vi "Call Async Do.vi"(10 "Async Methods Actor in":refnum<class "Async Methods Actor.lvclass">, 11 "Message in":refnum<class "Message.lvclass">) -> (0 "error out":errorcluster, 2 "Async Methods Actor out":refnum<class "Async Methods Actor.lvclass">)   [LabVIEW 2021, in "Async Methods Actor.lvlib" / "Async Methods Actor.lvclass"]
uses:
  Async Methods Actor.lvclass
  <vilib>/ActorFramework/Message/Message.lvclass
  C:/Program Files/National Instruments/LabVIEW 2021/vi.lib/ActorFramework/Actor/Actor.lvclass
  Async Methods Actor.lvclass/Async Methods Actor.ctl
  VI Refnums Map Value.ctl
  Async Call Method.ctl
  VI Refnum Lifetime.ctl
  Async Methods Actor Messages/Async Message/Async Message.lvclass
  Async Methods Actor Messages/Async Message/Async Message.lvclass/Async Message.ctl
  Async Methods Actor Messages/Async Message/Read Async Call Method.vi
  Async Methods Actor Messages/Async Message/Read VI Refnum Lifetime.vi
  Write Async Message Execution Status Map.vi
  Async Methods Actor Messages/Async Message/Read FQN.vi
  Write Async Message Execution Status Map.vi/3adbf29e-89d7-4ecb-a2bd-8a8b89d527f8.vi
  Get VI FQN.vi
  <vilib>/ActorFramework/Actor/Actor.lvclass
  C:/Projects/Async Methods Actor/Async Methods Actor/Async Methods Actor/Async Methods Actor.lvclass
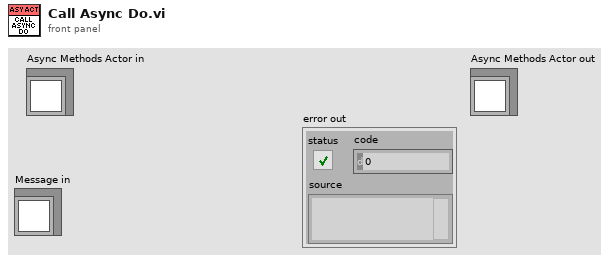
[diagram p1: front panel]
types:
  T1 = typedef "Async Methods Actor.lvlib/Async Methods Actor.lvclass/VI Refnums Map Value.ctl" = cluster{"Async Call Method":T2, "VI Refnum Lifecycle":T3, "Message Path":path}
  T2 = typedef "Async Methods Actor.lvlib/Async Methods Actor.lvclass/Async Call Method.ctl" = enum16{"Call and Collect", "Call and Forget"}
  T3 = typedef "Async Methods Actor.lvlib/Async Methods Actor.lvclass/VI Refnum Lifetime.ctl" = enum16{"Destroy on Exit", "Destroy on Actor Exit", "Leak"}
  T4 = typedef "Async Methods Actor.lvlib/Async Methods Actor.lvclass/VI Refnums Map.ctl" = map{refnum<vi>, T1}
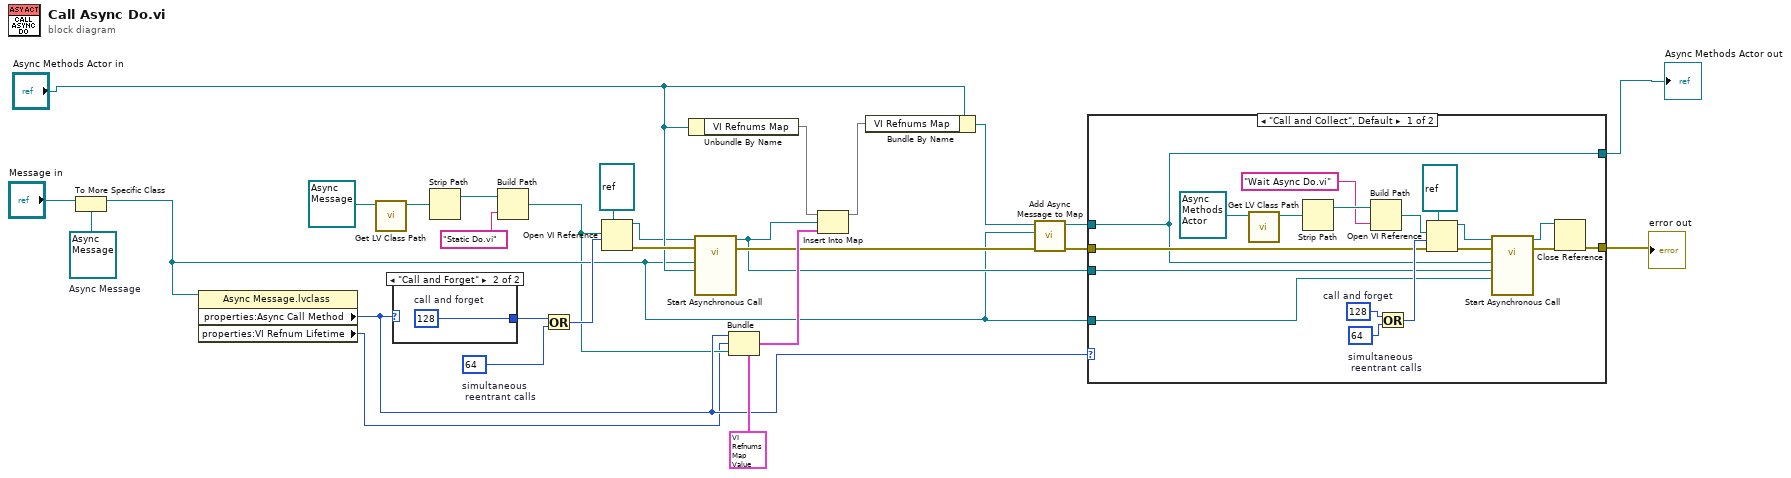
[diagram p0: block diagram]
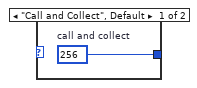
[diagram p3: hidden frame]
diagram:
  w25 = refnum<class "Async Message.lvclass"> refnum  # Async Message
  w23 = 64  # simultaneous  reentrant calls
  n1 = To More Specific Class(target class=w25, reference="Message in") -> (specific class reference=w3:refnum<class "Async Message.lvclass">)  [unwired: 1 in, 1 out]
  n2 = property class="Async Message.lvclass"(reference=w3) -> ("properties:Async Call Method"=w10:T2, "properties:VI Refnum Lifetime"=w1:T3)  [unwired: 1 in, 2 out]
  n3 = call <vilib>:"Get LV Class Path.vi"("object"=refnum<class "Async Message.lvclass"> refnum ("Async Actor.lvlib:Async Message.lvclass")) -> ("class path"=w20:path)  [unwired: 9 in, 1 out]
  n4 = case shown="\"Call and Forget\"" w10 {
    tunnel: [w29 w30] -> w26
    frame "Call and Collect", Default {
      w29 = 256  # call and collect
    }
    frame "Call and Forget" {
      w30 = 128  # call and forget
    }
  }
  n5 = Strip Path(path=w20) -> (stripped path=w5:path)  [unwired: 1 out]
  n6 = Build Path(base path=w5, name or relative path="Static Do.vi") -> (appended path=w2:path)
  n7 = Or(x=w26, y=w23) -> (x .or. y?=w22:i32)
  n8 = Open VI Reference(type specifier VI Refnum (for type only)=refnum<vi> refnum, vi path=w2, options=w22) -> (vi reference=w4:refnum<vi>, error out=w18:errorcluster)  [unwired: 3 in]
  n9 = Unbundle By Name("Async Methods Actor in") -> ("VI Refnums Map"=w27:T4)
  n10 = call-by-ref "Start Asynchronous Call"(reference=w4, error in=w18, "Actor in"="Async Methods Actor in", "Async Message"=w3) -> (reference out=w6:refnum<vi>, error out=w14:errorcluster)  [unwired: 8 in, 2 out]
  n11 = Bundle(cluster=T1 {"Async Call Method"=enum."Call and Collect", "VI Refnum Lifecycle"=enum."Destroy on Exit", "Message Path"=path ""} ("VI Refnums Map Value"), "Async Call Method"=w10, "VI Refnum Lifecycle"=w1, "Message Path"=w2) -> (w15:T1)
  n12 = Insert Into Map(map in=w27, key=w6, value=w15) -> (map out=w28:T4)  [unwired: 2 out]
  n13 = Bundle By Name(cluster="Async Methods Actor in", "VI Refnums Map"=w28) -> (w12:refnum<class "Async Methods Actor.lvclass">)
  n14 = call "Add Async Message to Map.vi"("error in (no error)"=w14, "Message"=w3, "Async Methods Actor in"=w12) -> ("error out"=w13:errorcluster, "Async Methods Actor out"=w11:refnum<class "Async Methods Actor.lvclass">)  [unwired: 7 in]
  n15 = case shown="\"Call and Collect\", Default" w10 {
    tunnel: [w37 w50] -> w17
    tunnel: w6 -> [w36 _]
    tunnel: w13 -> [w35 w50]
    tunnel: w11 -> [w34 w49]
    tunnel: [w34 w49] -> w8
    tunnel: w3 -> [w31 _]
    frame "Call and Collect", Default {
      w41 = 64  # simultaneous  reentrant calls
      w42 = 128  # call and forget
      n16 = call <vilib>:"Get LV Class Path.vi"("object"=refnum<class "Async Methods Actor.lvclass"> refnum ("Async Methods Actor.lvlib:Async Methods Actor.lvclass")) -> ("class path"=w46:path)  [unwired: 9 in, 1 out]
      n17 = Strip Path(path=w46) -> (stripped path=w48:path)  [unwired: 1 out]
      n18 = Build Path(base path=w48, name or relative path="Wait Async Do.vi") -> (appended path=w44:path)
      n19 = Or(x=w42, y=w41) -> (x .or. y?=w40:i32)
      n20 = Open VI Reference(type specifier VI Refnum (for type only)=refnum<vi> refnum, vi path=w44, options=w40, error in (no error)=w35) -> (vi reference=w43:refnum<vi>, error out=w45:errorcluster)  [unwired: 2 in]
      n21 = call-by-ref "Start Asynchronous Call"(reference=w43, error in=w45, "Async Message"=w31, "VI Refnum"=w36, "Async Methods Actor in"=w34) -> (reference out=w38:refnum<vi>, error out=w39:errorcluster)  [unwired: 7 in, 2 out]
      n22 = Close Reference(reference=w38, error in (no error)=w39) -> (error out=w37:errorcluster)
    }
    frame "Call and Forget" {
    }
  }
  "error out" <- w17
  "Async Methods Actor out" <- w8
